vi "Manual Mode.vi"() -> ()   [LabVIEW 2015]
uses:
  CAN Communication/Gas/Typedefs/Valves.ctl
  CAN Communication/Peltier/Typedefs/Peltier Temperature Sensors.ctl
  CAN Communication/Gas/Gas.lvclass
  Common/Buffers/Snapshot/Snapshot.lvclass
  CAN Communication/Peltier/Peltier.lvclass
panel:
  in  "PSI":dbl
  in  "Regulate Pressure":bool
  in  "Dump":bool
  out "Test Leak Rate (PSI/s)":dbl format="%#.2g"
  out "Pelt":errorcluster caption="Peltier Board Errors"
  out "TS5":dbl caption="Temp Sensor 5" format="%#.2g"
  out "TS4":dbl caption="Temp Sensor 4" format="%#.2g"
  out "TS3":dbl caption="Temp Sensor 3" format="%#.2g"
  out "TS2":dbl caption="Temp Sensor 2" format="%#.2g"
  out "TS1":dbl caption="Temp Sensor 1" format="%#.2g"
  in  "Pelt":bool
  out "DAQ Errors":errorcluster
  out "Gas Pressure EX (PSI)":dbl format="%#.2g"
  out "Gas Board Errors":errorcluster
  in  "Valves":T1=52 items=["GV1"=33, "GV2"=34, "GV3"=35, "GV4"=36, "GV5"=37, "GV6"=38, "GV7"=39, "GV8"=40, "GV9"=41, "GV10"=42, "GV11"=43, "LV3"=51, "LV4"=52]
  in  "Gas Pump":bool
  in  "LV4":bool
  in  "LV3":bool
  in  "GV10":bool
  in  "GV9":bool
  in  "GV8":bool
  in  "GV7":bool
  in  "GV6":bool
  in  "GV5":bool
  in  "GV4":bool
  out "Control Block Error":errorcluster
  in  "SV1":bool
  in  "GV4":bool
  in  "GV3":bool
  out "Gas Pressure GC (PSI)":dbl format="%#.2g"
  in  "OK Button":bool
  in  "GV3":bool
  in  "GV2":bool
  in  "GV1":bool
  in  "Vacuum":bool
  in  "GV2":bool
  in  "GV1":bool
  in  "SV2":bool
  out "Test Pressure (PSI)":dbl format="%#.2g"
  # "Manual Mode"
  # "Pressure Readings"
  # "Control Block"
  # "Gas Board"
  # "Peltier Board"
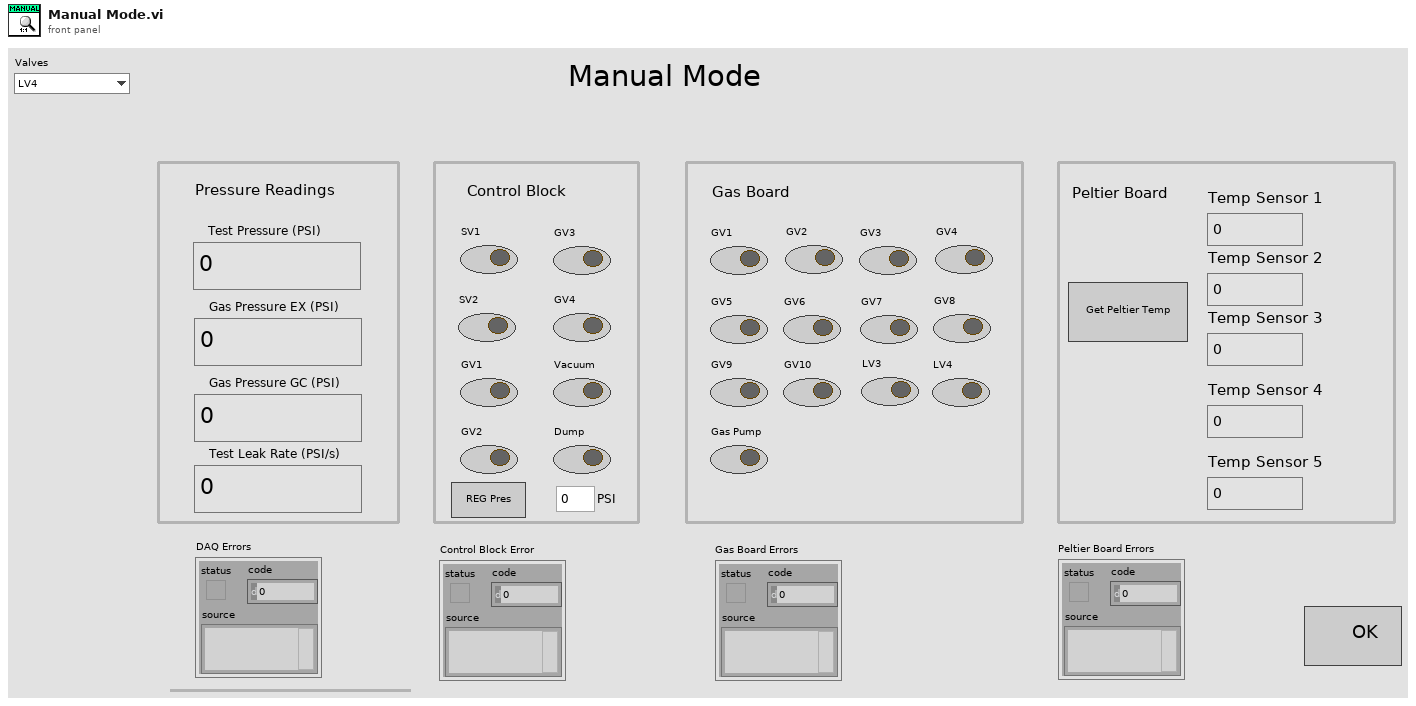
[diagram p1: front panel]
types:
  T1 = typedef "Gas.lvclass/Valves.ctl" = u16
  T2 = typedef "Gas.lvclass/Session Handle.ctl" = refnum<data-value>
  T3 = typedef "Snapshot.lvclass/Session Handle.ctl" = refnum<data-value>
  T4 = typedef "LVStringsAndValuesArrayTypeDef_U16.ctl" = cluster{"String":string, "Value":u16}[]
  T5 = typedef "Peltier.lvclass/Peltier Temperature Sensors.ctl" = u16
  T6 = typedef "Peltier.lvclass/Session Handle.ctl" = refnum<data-value>
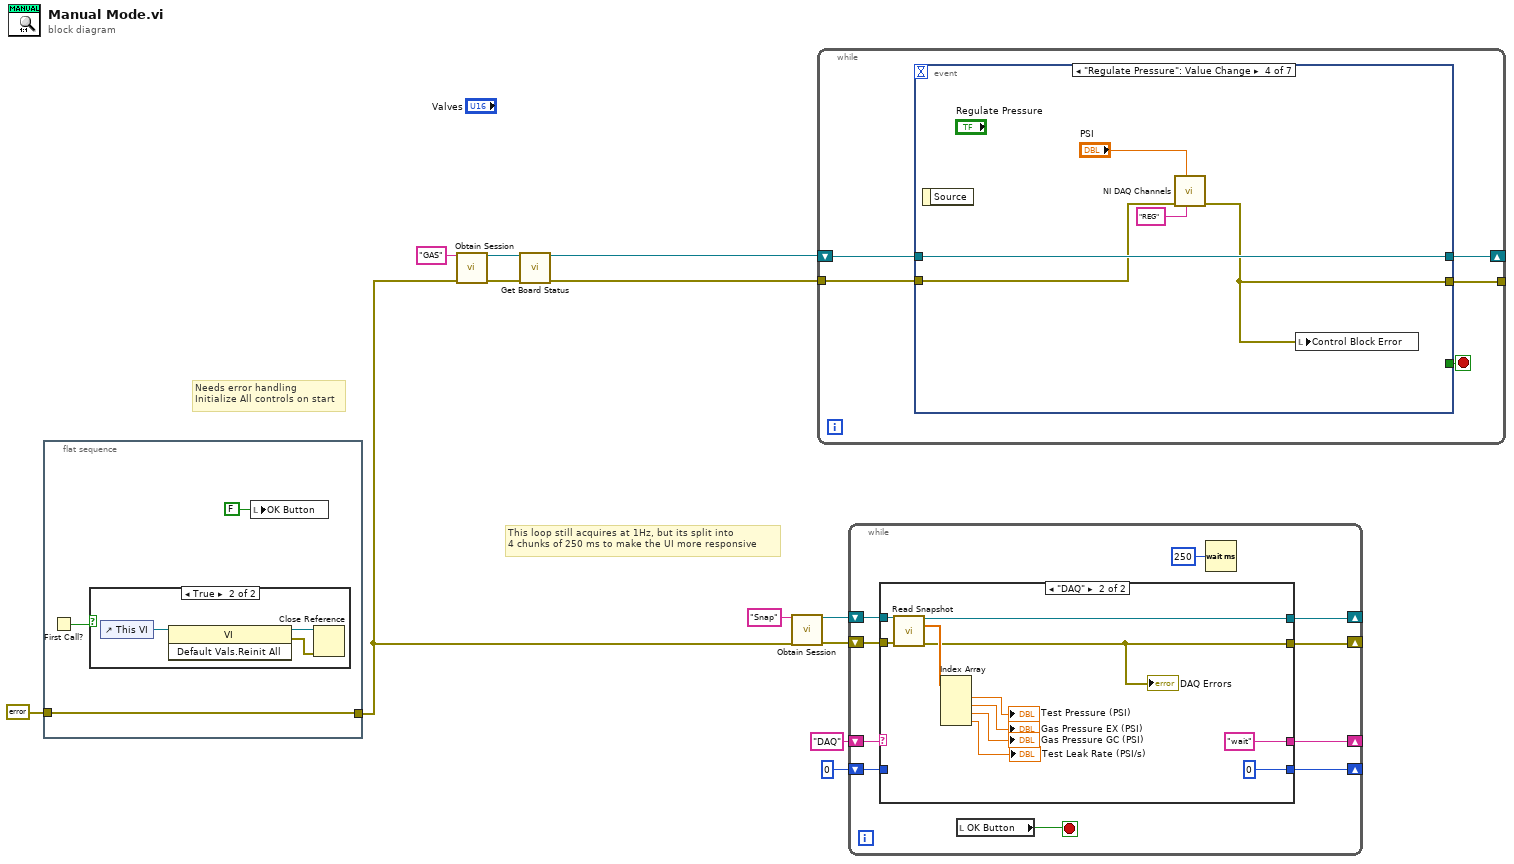
[diagram p0: block diagram]
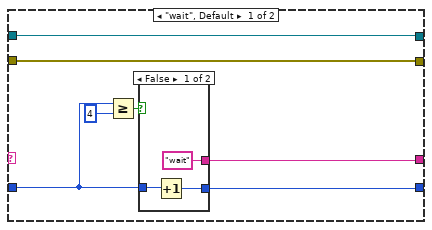
[diagram p2: hidden frame]
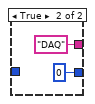
[diagram p3: hidden frame]
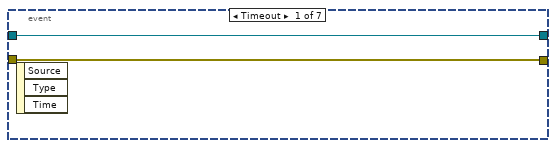
[diagram p5: hidden frame]
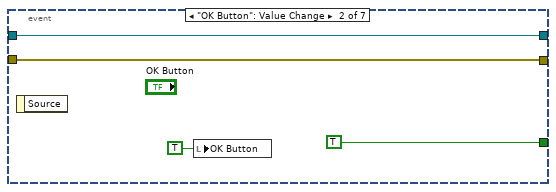
[diagram p6: hidden frame]
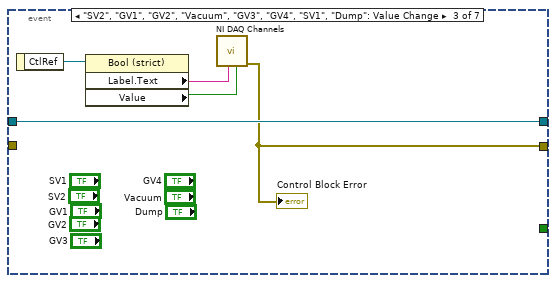
[diagram p7: hidden frame]
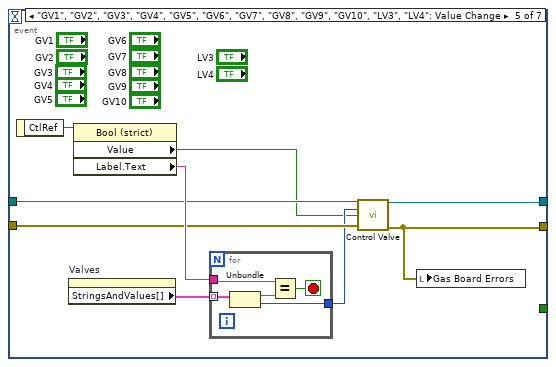
[diagram p8: hidden frame]
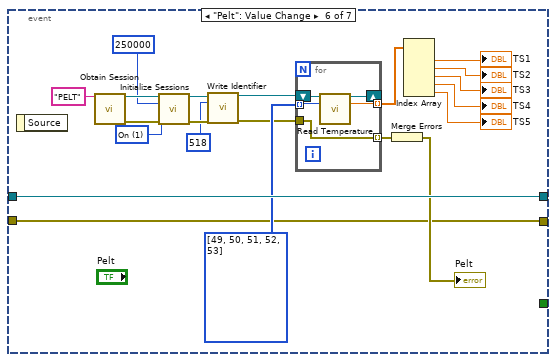
[diagram p9: hidden frame]
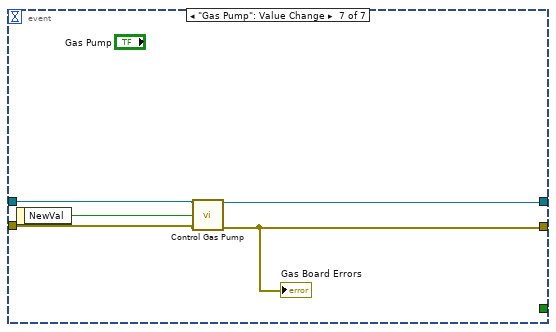
[diagram p10: hidden frame]
diagram:
  # "This loop still acquires at 1Hz, but its split into\n4 chunks of 250 ms to make the UI more responsive"
  # "Needs error handling\nInitialize All controls on start"
  n1 = flat-sequence {
    tunnel: errorcluster {"status"=FALSE, "code"=0, "source"=""} ("error in (no error)") -> [w14]
    tunnel: [w14] -> w1
    frame #0 {
      n2 = First Call?() -> (First Call?: T/F=w13:bool)
      n3 = case shown="True" w13 {
        frame False {
        }
        frame True {
          n4 = control-ref of="This VI"() -> (w18:refnum<vi>)
          n5 = invoke class="VI" method="Default Vals.Reinit All"(reference=w18) -> (reference out=w16:refnum<vi>, error out=w17:errorcluster)  [unwired: 2 in, 1 out]
          n6 = Close Reference(reference=w16, error in (no error)=w17) -> ()  [unwired: 1 out]
        }
      }
      n7 = local write "OK Button"(FALSE ("OK Button")) -> ()
    }
  }
  n8 = call "Obtain Session.vi"("Session  Name ()"="GAS", "error in (no error)"=w1) -> ("Session Handle"=w10:T2, "error out"=w9:errorcluster)  [unwired: 12 in]
  n9 = call "Get Board Status.vi"("Session Handle in"=w10, "error in (no error)"=w9) -> ("Session Handle out"=w8:T2, "error out"=w7:errorcluster)  [unwired: 11 in, 1 out]
  n10 = call "Obtain Session.vi"("Session  Name ()"="Snap", "error in (no error)"=w1) -> ("Session Handle"=w5:T3, "error out"=w4:errorcluster)  [unwired: 12 in]
  n11 = while {
    shift-right: [w21] -> _
    shift-left: w8 -> [w23]
    tunnel: w7 -> [w22]
    tunnel: [w20] -> _
    stop <- w19 stop-if-true
    n12 = event shown="[3] \"Regulate Pressure\": Value Change" {
      selector: _ -> [_ _ _ _ _ _ _]
      dyn-events: _ -> [_ _ _ _ _ _ _]
      timeout: _ -> [_ _ _ _ _ _ _]
      tunnel: w23 -> [w25 w29 w34 w39 w44 w74 w84]
      tunnel: w22 -> [w24 w28 _ w37 w45 w54 w82]
      tunnel: [w25 w29 w34 w39 w41 w74 w83] -> w21
      tunnel: [w24 w28 w30 w35 w40 w54 w80] -> w20
      tunnel: [_ TRUE ("OK Button") _ _ _ _ _] -> w19
      event Timeout {
        n13 = event-data() -> ()  [unwired: 1 in, 3 out]
      }
      event "OK Button": Value Change {
        n14 = event-data() -> ()  [unwired: 1 in, 1 out]
        n15 = local write "OK Button"(TRUE ("OK Button")) -> ()
      }
      event "SV2", "GV1", "GV2", "Vacuum", "GV3", "GV4", "SV1", "Dump": Value Change {
        n16 = event-data() -> ("CtlRef"=w33:refnum<vi>)  [unwired: 1 in]
        n17 = property class="Bool (strict)"(reference=w33) -> ("Label.Text"=w32:string, "Value"=w31:bool)  [unwired: 1 in, 2 out]
        n18 = call "NI DAQ Channels.vi"("Control"=w31, "Channel"=w32) -> ("error out"=w30:errorcluster)  [unwired: 8 in, 1 out]
        "Control Block Error" <- w30
      }
      event "Regulate Pressure": Value Change {
        n19 = event-data() -> ()  [unwired: 1 in, 1 out]
        n20 = call "NI DAQ Channels.vi"("Channel"="REG", "AO Data"="PSI", "error in (no error)"=w37) -> ("error out"=w35:errorcluster)  [unwired: 7 in, 1 out]
        n21 = local write "Control Block Error"(w35) -> ()
      }
      event "GV1", "GV2", "GV3", "GV4", "GV5", "GV6", "GV7", "GV8", "GV9", "GV10", "LV3", "LV4": Value Change {
        n22 = event-data() -> ("CtlRef"=w47:refnum<vi>)  [unwired: 1 in]
        n23 = property on="Valves" class="Ring (strict)"() -> ("StringsAndValues[]"=w48:T4)  [unwired: 2 in, 2 out]
        n24 = property class="Bool (strict)"(reference=w47) -> ("Value"=w42:bool, "Label.Text"=w46:string)  [unwired: 1 in, 2 out]
        n25 = for {
          tunnel: w48 -> [w53] mode=indexing
          tunnel: w46 -> [w51]
          tunnel: [w49] -> w43
          stop <- w50 stop-if-true
          n26 = Unbundle(w53) -> ("String"=w52:string, "Value"=w49:u16)
          n27 = Equal?(x=w51, y=w52) -> (x = y?=w50:bool)
        }
        n28 = call "Control Valve.vi"("Session Handle in"=w44, "Valves"=w43, "Energize?"=w42, "error in (no error)"=w45) -> ("Session Handle out"=w41:T2, "error out"=w40:errorcluster)  [unwired: 9 in, 1 out]
        n29 = local write "Gas Board Errors"(w40) -> ()
      }
      event "Pelt": Value Change {
        w65 = T5[] [49, 50, 51, 52, 53] items=["PTS1"=49, "PTS2"=50, "PTS3"=51, "PTS4"=52, "PTS5"=53, "PTS6"=54]
        w69 = u32 1 items=["Off", "On"] ("Termination")
        n30 = event-data() -> ()  [unwired: 1 in, 1 out]
        n31 = call "Obtain Session.vi"("Session  Name ()"="PELT") -> ("Session Handle"=w72:T6, "error out"=w71:errorcluster)  [unwired: 13 in]
        n32 = call "Initialize Sessions.vi"("Session Handle"=w72, "Baud Rate"=u32 250000, "Termination"=w69, "error in (no error)"=w71) -> ("Session Handle Out"=w68:T6, "error out"=w67:errorcluster)  [unwired: 10 in]
        n33 = call "Write Identifier.vi"("Session Handle In"=w68, "identifier"=u16 518, "error in (no error)"=w67) -> ("Session Handle Out"=w64:T6, "error out"=w63:errorcluster)  [unwired: 11 in]
        n34 = for {
          shift-right: [w78] -> _
          shift-left: w64 -> [w79]
          tunnel: [w77] -> w62 mode=indexing
          tunnel: w65 -> [w76] mode=indexing
          tunnel: w63 -> [w75]
          tunnel: [w75] -> w61 mode=indexing
          n35 = call "Read Temperature.vi"("Session Handle"=w79, "Pelt Temp Sensors"=w76) -> ("Session Handle Out"=w78:T6, "Temperature"=w77:dbl)  [unwired: 11 in, 1 out]
        }
        n36 = Merge Errors(w61) -> (→"Pelt":errorcluster)
        n37 = Index Array(array=w62) -> (element #1=→"TS1":dbl, element #2=→"TS2":dbl, element #3=→"TS3":dbl, element #4=→"TS4":dbl, element #5=→"TS5":dbl)  [unwired: 5 in]
      }
      event "Gas Pump": Value Change {
        n38 = event-data() -> ("NewVal"=w81:bool)  [unwired: 1 in]
        n39 = call "Control Gas Pump.vi"("Session Handle in"=w84, "On?"=w81, "error in (no error)"=w82) -> ("Session Handle out"=w83:T2, "error out"=w80:errorcluster)  [unwired: 10 in, 1 out]
        "Gas Board Errors" <- w80
      }
    }
  }
  n40 = while {
    shift-right: [w91] -> _
    shift-left: w5 -> [w92]
    shift-right: [w90] -> _
    shift-left: w4 -> [w93]
    shift-right: [w88] -> _
    shift-left: "DAQ" -> [w89]
    shift-right: [w87] -> _
    shift-left: 0 -> [w86]
    stop <- w94 stop-if-true
    n41 = case shown="\"DAQ\"" w89 {
      tunnel: w93 -> [w100 w117]
      tunnel: w92 -> [w101 w116]
      tunnel: [w101 w115] -> w91
      tunnel: [w100 w108] -> w90
      tunnel: [w95 "wait"] -> w88
      tunnel: [w96 0] -> w87
      tunnel: w86 -> [w97 _]
      frame "wait", Default {
        n42 = Greater Or Equal?(x=w97, y=4) -> (x >= y?=w98:bool)
        n43 = case shown="False" w98 {
          tunnel: w97 -> [w104 _]
          tunnel: [w103 0] -> w96
          tunnel: ["wait" "DAQ"] -> w95
          frame False {
            n44 = Increment(x=w104) -> (x+1=w103:i32)
          }
          frame True {
          }
        }
      }
      frame "DAQ" {
        n45 = call "Read Snapshot.vi"("Session Handle in"=w116, "error in (no error)"=w117) -> ("Session Handle out"=w115:T3, "Buffer"=w114:dbl[], "error out"=w108:errorcluster)  [unwired: 11 in]
        "DAQ Errors" <- w108
        n46 = Index Array(array=w114) -> (element #1=→"Test Pressure (PSI)":dbl, element #2=→"Gas Pressure EX (PSI)":dbl, element #3=→"Gas Pressure GC (PSI)":dbl, element #4=→"Test Leak Rate (PSI/s)":dbl)  [unwired: 4 in]
      }
    }
    n47 = local read "OK Button"() -> (w94:bool)
    n48 = Wait (ms)(milliseconds to wait=u32 250) -> ()  [unwired: 1 out]
  }
